vi "SequenceIndexCheck.vi"(8 "error in (no error)":errorcluster, 9 "OriginalName":string, 10 "SequenceIndex":refnum<class "SequenceIndex.lvclass">, 11 "VariableManager in":refnum<class "VariableManager.lvclass">) -> (0 "error out":errorcluster, 1 "RejectMessage":string, 2 "Pass":bool=TRUE, 3 "VariableManager out":refnum<class "VariableManager.lvclass">)   [LabVIEW 2013, in "VariableManager.lvclass"]
doc: "Check the given sequence index definition before adding to database.\n\nReturn true if the given sequence index passes all tests.\nReturn false if the given sequence index fails some tests.\nRejectMessage can be used to identify the failed tests. \n\nThe following will make a sequence index definition fails the test:\n1. The difinition has an empty name\n2. Steps is less than 1\n3. The name is already used by another sequence index. Providing OriginalName will bypass the check against the given OriginalName\n4. The name is already used by another variable.\n5. The name begins with number.\n6. The name is t or f (reserved variable name)"
uses:
  VariableManager.lvclass
  SequenceIndex/SequenceIndex.lvclass
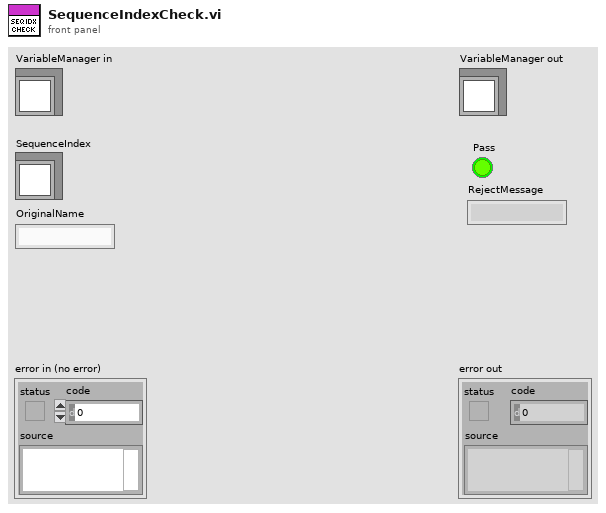
[diagram p1: front panel]
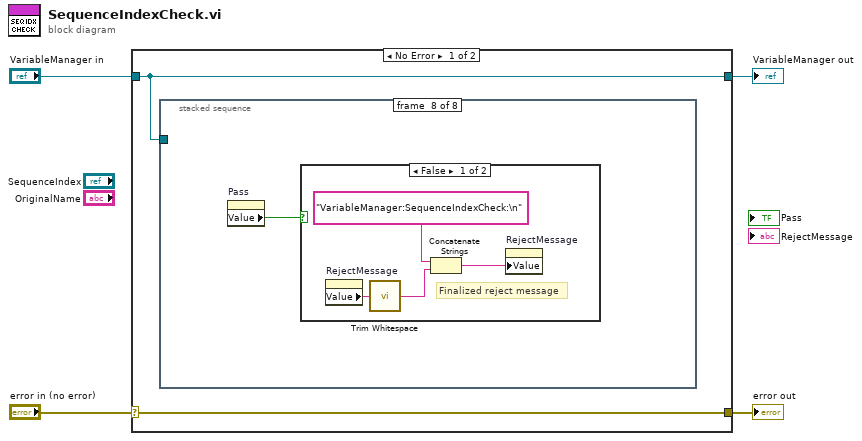
[diagram p0: block diagram]
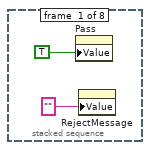
[diagram p2: hidden frame]
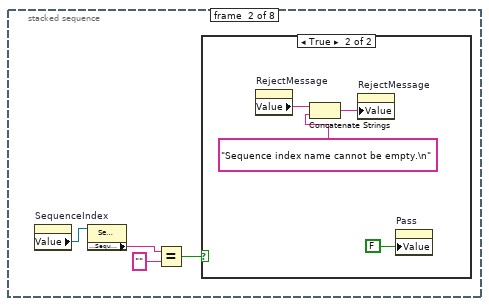
[diagram p3: hidden frame]
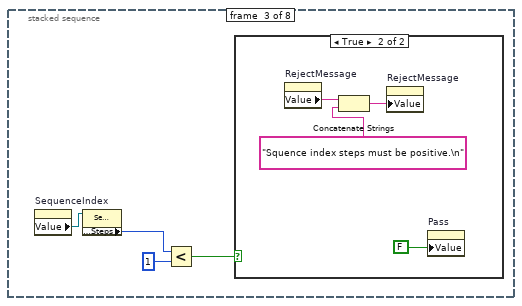
[diagram p5: hidden frame]
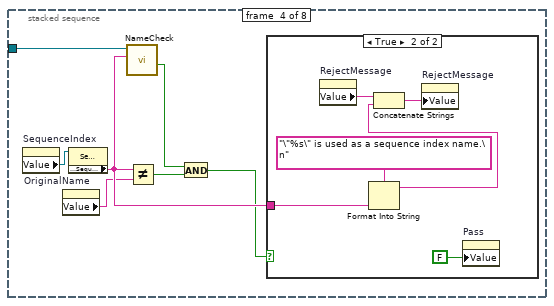
[diagram p7: hidden frame]
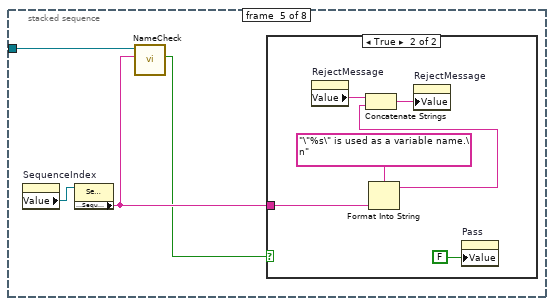
[diagram p9: hidden frame]
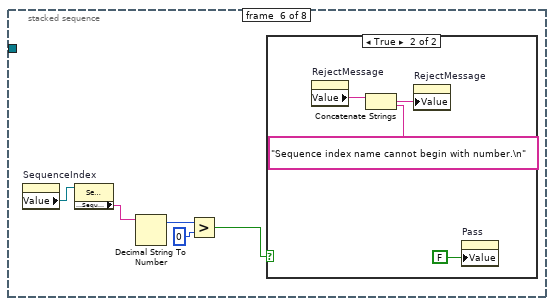
[diagram p11: hidden frame]
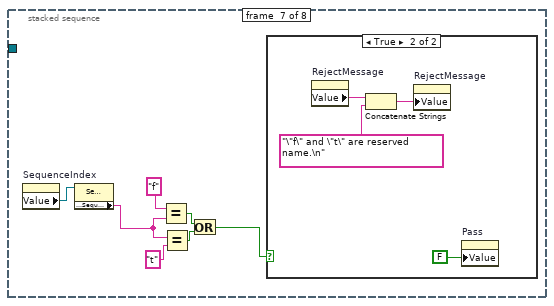
[diagram p13: hidden frame]
diagram:
  n1 = case shown="No Error" "error in (no error)" {
    selector: "error in (no error)" -> [w6 w74]
    tunnel: [w6 w74] -> w3
    tunnel: [w5 w73] -> w1
    tunnel: "VariableManager in" -> [w5 w73]
    frame No Error {
      n2 = stacked-sequence {
        tunnel: w5 -> [_ _ _ w25 w38 _ _ _]
        frame #0 {
          n3 = property on="Pass" class="Bool (strict)"("Value"=TRUE ("Pass")) -> ()  [unwired: 2 in, 2 out]
          n4 = property on="RejectMessage" class="Str"("Value"="") -> ()  [unwired: 2 in, 2 out]
        }
        frame #1 {
          n5 = property on="SequenceIndex" class="LVClassControl (strict)"() -> ("Value"=w10:refnum<class "SequenceIndex.lvclass">)  [unwired: 2 in, 2 out]
          n6 = property class="SequenceIndex.lvclass"(reference=w10) -> ("Accessors:SequenceIndexName"=w12:string)  [unwired: 1 in, 2 out]
          n7 = Equal?(x=w12, y="") -> (x = y?=w9:bool)
          n8 = case shown="True" w9 {
            frame False {
            }
            frame True {
              n9 = property on="RejectMessage" class="Str"() -> ("Value"=w15:string)  [unwired: 2 in, 2 out]
              n10 = Concatenate Strings(w15, "Sequence index name cannot be empty.\n") -> (w14:string)
              n11 = property on="RejectMessage" class="Str"("Value"=w14) -> ()  [unwired: 2 in, 2 out]
              n12 = property on="Pass" class="Bool (strict)"("Value"=FALSE ("Pass")) -> ()  [unwired: 2 in, 2 out]
            }
          }
        }
        frame #2 {
          n13 = property on="SequenceIndex" class="LVClassControl (strict)"() -> ("Value"=w20:refnum<class "SequenceIndex.lvclass">)  [unwired: 2 in, 2 out]
          n14 = property class="SequenceIndex.lvclass"(reference=w20) -> ("Accessors:Steps"=w19:u32)  [unwired: 1 in, 2 out]
          n15 = Less?(x=w19, y=u32 1) -> (x < y?=w17:bool)
          n16 = case shown="True" w17 {
            frame False {
            }
            frame True {
              n17 = property on="RejectMessage" class="Str"() -> ("Value"=w23:string)  [unwired: 2 in, 2 out]
              n18 = Concatenate Strings(w23, "Squence index steps must be positive.\n") -> (w22:string)
              n19 = property on="RejectMessage" class="Str"("Value"=w22) -> ()  [unwired: 2 in, 2 out]
              n20 = property on="Pass" class="Bool (strict)"("Value"=FALSE ("Pass")) -> ()  [unwired: 2 in, 2 out]
            }
          }
        }
        frame #3 {
          n21 = property on="SequenceIndex" class="LVClassControl (strict)"() -> ("Value"=w28:refnum<class "SequenceIndex.lvclass">)  [unwired: 2 in, 2 out]
          n22 = property on="OriginalName" class="Str"() -> ("Value"=w29:string)  [unwired: 2 in, 2 out]
          n23 = property class="SequenceIndex.lvclass"(reference=w28) -> ("Accessors:SequenceIndexName"=w30:string)  [unwired: 1 in, 2 out]
          n24 = call-dynamic "NameCheck.vi"("Name"=w30, "VariableManager in"=w25) -> ("UsedAsSequenceIndex"=w26:bool)  [unwired: 6 in, 3 out]
          n25 = Not Equal?(x=w30, y=w29) -> (x != y?=w31:bool)
          n26 = And(x=w26, y=w31) -> (x .and. y?=w27:bool)
          n27 = case shown="True" w27 {
            tunnel: w30 -> [_ w37]
            frame False {
            }
            frame True {
              n28 = property on="RejectMessage" class="Str"() -> ("Value"=w34:string)  [unwired: 2 in, 2 out]
              n29 = Format Into String(format string="\"%s\" is used as a sequence index name.\n", w37) -> (resulting string=w32:string)  [unwired: 2 in, 1 out]
              n30 = Concatenate Strings(w34, w32) -> (w33:string)
              n31 = property on="RejectMessage" class="Str"("Value"=w33) -> ()  [unwired: 2 in, 2 out]
              n32 = property on="Pass" class="Bool (strict)"("Value"=FALSE ("Pass")) -> ()  [unwired: 2 in, 2 out]
            }
          }
        }
        frame #4 {
          n33 = property on="SequenceIndex" class="LVClassControl (strict)"() -> ("Value"=w40:refnum<class "SequenceIndex.lvclass">)  [unwired: 2 in, 2 out]
          n34 = property class="SequenceIndex.lvclass"(reference=w40) -> ("Accessors:SequenceIndexName"=w41:string)  [unwired: 1 in, 2 out]
          n35 = call-dynamic "NameCheck.vi"("Name"=w41, "VariableManager in"=w38) -> ("UsedAsVariable"=w39:bool)  [unwired: 6 in, 3 out]
          n36 = case shown="True" w39 {
            tunnel: w41 -> [_ w47]
            frame False {
            }
            frame True {
              n37 = property on="RejectMessage" class="Str"() -> ("Value"=w44:string)  [unwired: 2 in, 2 out]
              n38 = Format Into String(format string="\"%s\" is used as a variable name.\n", w47) -> (resulting string=w42:string)  [unwired: 2 in, 1 out]
              n39 = Concatenate Strings(w44, w42) -> (w43:string)
              n40 = property on="RejectMessage" class="Str"("Value"=w43) -> ()  [unwired: 2 in, 2 out]
              n41 = property on="Pass" class="Bool (strict)"("Value"=FALSE ("Pass")) -> ()  [unwired: 2 in, 2 out]
            }
          }
        }
        frame #5 {
          n42 = property on="SequenceIndex" class="LVClassControl (strict)"() -> ("Value"=w52:refnum<class "SequenceIndex.lvclass">)  [unwired: 2 in, 2 out]
          n43 = property class="SequenceIndex.lvclass"(reference=w52) -> ("Accessors:SequenceIndexName"=w49:string)  [unwired: 1 in, 2 out]
          n44 = Decimal String To Number(string=w49) -> (offset past number=w50:i32)  [unwired: 2 in, 1 out]
          n45 = Greater?(x=w50, y=0) -> (0:w48:bool)
          n46 = case shown="True" w48 {
            frame False {
            }
            frame True {
              n47 = property on="RejectMessage" class="Str"() -> ("Value"=w55:string)  [unwired: 2 in, 2 out]
              n48 = Concatenate Strings(w55, "Sequence index name cannot begin with number.\n") -> (w54:string)
              n49 = property on="RejectMessage" class="Str"("Value"=w54) -> ()  [unwired: 2 in, 2 out]
              n50 = property on="Pass" class="Bool (strict)"("Value"=FALSE ("Pass")) -> ()  [unwired: 2 in, 2 out]
            }
          }
        }
        frame #6 {
          n51 = property on="SequenceIndex" class="LVClassControl (strict)"() -> ("Value"=w63:refnum<class "SequenceIndex.lvclass">)  [unwired: 2 in, 2 out]
          n52 = property class="SequenceIndex.lvclass"(reference=w63) -> ("Accessors:SequenceIndexName"=w57:string)  [unwired: 1 in, 2 out]
          n53 = Equal?(x="f", y=w57) -> (x = y?=w59:bool)
          n54 = Equal?(x=w57, y="t") -> (x = y?=w60:bool)
          n55 = Or(x=w59, y=w60) -> (x .or. y?=w58:bool)
          n56 = case shown="True" w58 {
            frame False {
            }
            frame True {
              n57 = property on="RejectMessage" class="Str"() -> ("Value"=w66:string)  [unwired: 2 in, 2 out]
              n58 = Concatenate Strings(w66, "\"f\" and \"t\" are reserved name.\n") -> (w65:string)
              n59 = property on="RejectMessage" class="Str"("Value"=w65) -> ()  [unwired: 2 in, 2 out]
              n60 = property on="Pass" class="Bool (strict)"("Value"=FALSE ("Pass")) -> ()  [unwired: 2 in, 2 out]
            }
          }
        }
        frame #7 {
          n61 = property on="Pass" class="Bool (strict)"() -> ("Value"=w68:bool)  [unwired: 2 in, 2 out]
          n62 = case shown="False" w68 {
            frame False {
              # "Finalized reject message"
              n63 = property on="RejectMessage" class="Str"() -> ("Value"=w70:string)  [unwired: 2 in, 2 out]
              n64 = call <vilib>:"Trim Whitespace.vi"("string"=w70) -> ("trimmed string"=w71:string)  [unwired: 1 in]
              n65 = Concatenate Strings("VariableManager:SequenceIndexCheck:\n", w71) -> (w69:string)
              n66 = property on="RejectMessage" class="Str"("Value"=w69) -> ()  [unwired: 2 in, 2 out]
            }
            frame True {
            }
          }
        }
      }
    }
    frame Error {
    }
  }
  "error out" <- w3
  "VariableManager out" <- w1
